vi "Shortcut Menu Selection.vi"(8 "Error In":errorcluster, 9 "Tree Tag":string, 10 "Data":variant, 11 "State In":T1) -> (0 "Error Out":errorcluster, 3 "State Out":T1)   [LabVIEW 2017, in "Bookmark Manager.lvlib"]
uses:
  Bookmark Manager.lvlib
  Controls/State.ctl
  Controls/VI Bookmark.ctl
  Controls/VI Information.ctl
  Controls/Application Information.ctl
  Controls/Bookmarks Views.ctl
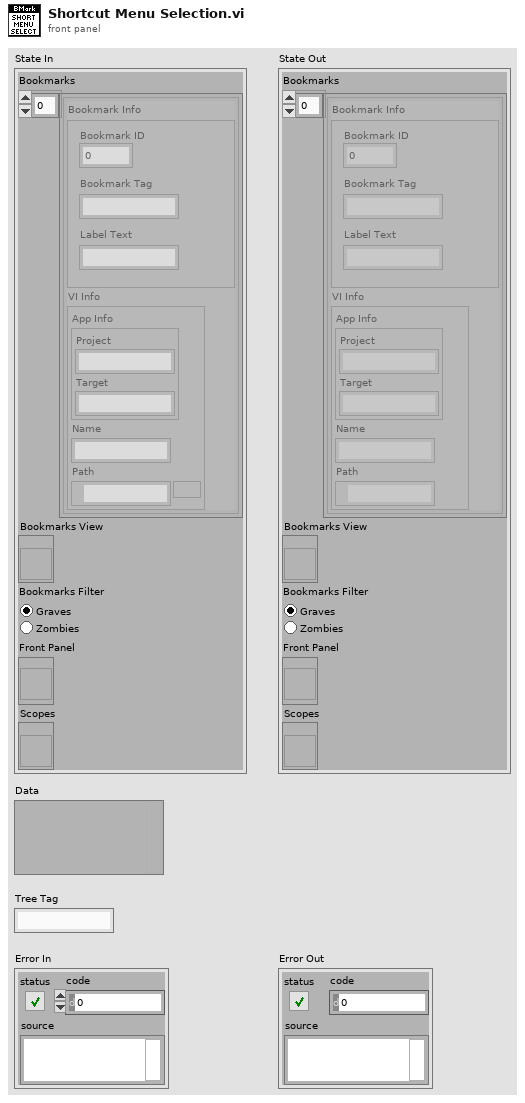
[diagram p1: front panel]
types:
  T1 = typedef "Bookmark Manager.lvlib/State.ctl" = cluster{"Bookmarks":T2[], "Bookmarks View":refnum<vi>, "Bookmarks Filter":T5, "Front Panel":refnum<vi>, "Scopes":refnum<vi>}
  T2 = typedef "Bookmark Manager.lvlib/VI Bookmark.ctl" = cluster{"Bookmark Info":cluster{"Bookmark ID":u32, "Bookmark Tag":string, "Label Text":string}, "VI Info":T3}
  T3 = typedef "Bookmark Manager.lvlib/VI Information.ctl" = cluster{"App Info":T4, "Name":string, "Path":path}
  T4 = typedef "Bookmark Manager.lvlib/Application Information.ctl" = cluster{"Project":string, "Target":string}
  T5 = typedef "Bookmark Manager.lvlib/Bookmarks Views.ctl" = enum32{"Graves", "Zombies"}
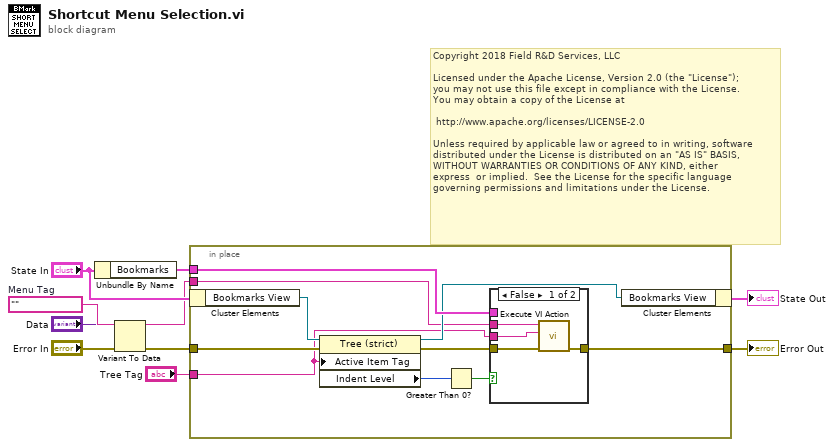
[diagram p0: block diagram]
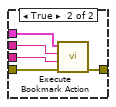
[diagram p2: hidden frame]
diagram:
  w5 = ""  # Menu Tag
  # "Copyright 2018 Field R&D Services, LLC\n\nLicensed under the Apache License, Version 2.0 (the \"License\");\nyou may not use this file except in compliance with the License.\nYou may obtain a copy of the License at\n\n\thttp://www.apache.org/licenses/LICENSE-2.0\n\nUnless required by applicable law or agreed to in writing, software\ndistributed under the License is distributed on an \"AS IS\" BASIS,\nWITHOUT WARRANTIES OR CONDITIONS OF ANY KIND, either \nexpress  or implied.  See the License for the specific language \ngoverning permissions and limitations under the License."
  n1 = Unbundle By Name("State In") -> ("Bookmarks"=w10:T2[])
  n2 = Variant To Data(error in="Error In", type=w5, Variant="Data") -> (data=w1:string, error out=w7:errorcluster)
  n3 = in-place {
    in-place-border: w7 -> [w16]
    in-place-border: [w19] -> w8
    in-place-border: w10 -> [w18]
    in-place-border: "Tree Tag" -> [w11]
    in-place-border: w1 -> [w12]
    n4 = in-place-cluster #1("State In") -> ("Bookmarks View"=w20:refnum<vi>)
    n5 = property class="Tree (strict)"(reference=w20, error in=w16, "Active Item Tag"=w11) -> (reference out=w17:refnum<vi>, error out=w15:errorcluster, "Indent Level"=w14:i32)
    n6 = Greater Than 0?(x=w14) -> (x > 0?=w13:bool)
    n7 = case shown="False" w13 {
      tunnel: w15 -> [w24 w29]
      tunnel: [w23 w28] -> w19
      tunnel: w18 -> [_ w27]
      tunnel: w12 -> [w22 w26]
      tunnel: w11 -> [w21 w25]
      frame False {
        n8 = call "Execute VI Action.vi"("Error In"=w24, "VI Tree Tag"=w21, "Menu Tag"=w22) -> ("Error Out"=w23:errorcluster)  [unwired: 8 in]
      }
      frame True {
        n9 = call "Execute Bookmark Action.vi"("Error In"=w29, "Tree Tag"=w25, "Menu Tag"=w26, "Bookmarks"=w27) -> ("Error Out"=w28:errorcluster)  [unwired: 7 in]
      }
    }
    n10 = in-place-cluster #1("Bookmarks View"=w17) -> (→"State Out":T1)
  }
  "Error Out" <- w8
